vi "WPI_GyroClose.vi"(8 "error in (no error)":errorcluster, 11 "GyroDevRef":T1={"DevStatus"={"status"=FALSE, "code"=0, "source"=""}, "Analog Channel"=enum."AI 1", "Gain (VoltsPerDegree/Second)"=0.0, "Gyro Type"=enum."Analog", "Handle"=0, "SPI Bus"=enum."Invalid", "Device Found"=FALSE, "Sample Rate"=1.0, "Calibrate On Open"=FALSE, "Offset"=0.0} {"Sample Rate" min=0.25 max=100.0 step=0.25}) -> (0 "error out":errorcluster)   [LabVIEW 2017]
doc: "Closes the reference to the gyroscope you specify. Use this VI to close each gyroscope reference that you open with the Open VI.\n\nThis software is licensed. Open the labview\\readme\\WPI Robotics Library Open Source License.txt file for more information."
uses:
  <vilib>/Rock Robotics/WPI/Gyro/WPI_GyroDevRef.ctl
  <vilib>/Rock Robotics/SystemInterfaces/AI/FPGA_AIChannel.ctl
  <vilib>/Rock Robotics/SystemInterfaces/spilib/spi_bus.ctl
  <vilib>/Rock Robotics/SystemInterfaces/AI/FPGA_AIGyroChannel.ctl
  <instrlib>/Sparkfun Atomic IMU/HAIOL/Sparkfun Atomic IMU.lvclass
  <instrlib>/Honeywell Compass HMC6343/HAIOL/Honeywell Compass HMC6343.lvclass
panel:
  # "Analog"
  # "XRS"
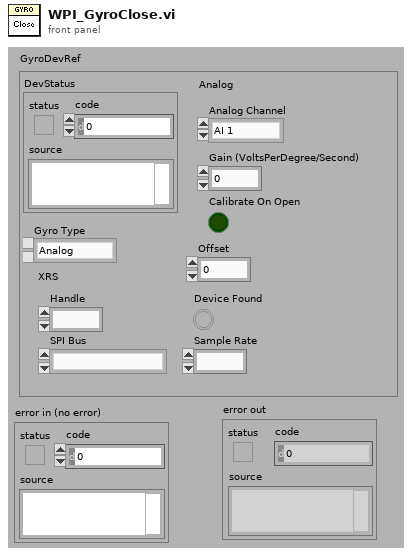
[diagram p1: front panel]
types:
  T1 = typedef "WPI_GyroDevRef.ctl" = cluster{"DevStatus":errorcluster, "Analog Channel":T2, "Gain (VoltsPerDegree/Second)":dbl, "Gyro Type":enum16{"Analog", "XRS450"}, "Handle":i32, "SPI Bus":T3, "Device Found":bool, "Sample Rate":dbl, "Calibrate On Open":bool, "Offset":dbl}
  T2 = typedef "FPGA_AIChannel.ctl" = enum8{"AI 0", "AI 1", "AI 2", "AI 3", "AI MXP 0", "AI MXP 1", "AI MXP 2", "AI MXP 3", "Invalid"}
  T3 = typedef "spi_bus.ctl" = enum16{"SPI On-Board, CS0", "SPI On-Board, CS1", "SPI On-Board, CS2", "SPI On-Board, CS3", "SPI MXP", "Invalid"}
  T4 = typedef "WPI_AnalogChannelDevRef.ctl" = cluster{"DevStatus":errorcluster, "Analog Channel":T2}
  T5 = typedef "FPGA_AIGyroChannel.ctl" = enum8{"AI 0", "AI 1", "Invalid"}
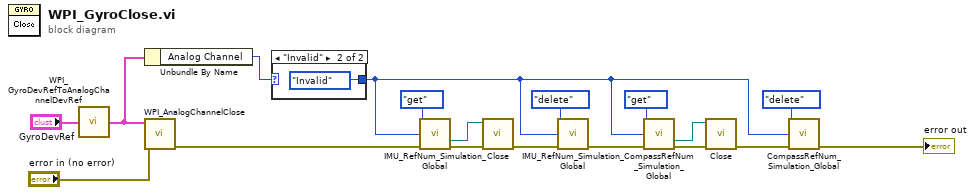
[diagram p0: block diagram]
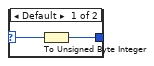
[diagram p2: hidden frame]
diagram:
  n1 = call <vilib>:"WPI_GyroDevRefToAnalogChannelDevRef.vi"("GyroDeviceRef"="GyroDevRef") -> ("AIDeviceRef"=w14:T4)  [unwired: 4 out]
  n2 = Unbundle By Name(w14) -> ("Analog Channel"=w13:T2)
  n3 = call <vilib>:"WPI_AnalogChannelClose.vi"("error in (no error)"="error in (no error)", "AIDeviceRef"=w14) -> ("error out"=w12:errorcluster)  [unwired: 9 out]
  n4 = case shown="\"Invalid\"" w13 {
    selector: w13 -> [w20 _]
    tunnel: [w19 FPGA_AIGyroChannel."Invalid" ("Analog Channel")] -> w3
    frame Default {
      n5 = To Unsigned Byte Integer(number=w20) -> (unsigned 8bit integer=w19:u8)
    }
    frame "Invalid" {
    }
  }
  n6 = call <vilib>:"IMU_RefNum_Simulation_Global.vi"("menu"=enum16{"set", "get", "delete"}."get", "Analog Channel"=w3, "error in (no error)"=w12) -> ("Sparkfun Atomic IMU Get"=w10:refnum<class "Sparkfun Atomic IMU.lvclass">, "error out"=w11:errorcluster)  [unwired: 11 in]
  n7 = call-dynamic "Close.vi"("error in (no error)"=w11, "Sparkfun Atomic IMU in"=w10) -> ("error out"=w8:errorcluster)  [unwired: 9 in]
  n8 = call <vilib>:"IMU_RefNum_Simulation_Global.vi"("menu"=enum16{"set", "get", "delete"}."delete", "Analog Channel"=w3, "error in (no error)"=w8) -> ("error out"=w7:errorcluster)  [unwired: 11 in, 1 out]
  n9 = call <vilib>:"CompassRefNum_Simulation_Global.vi"("menu"=enum16{"set", "get", "delete"}."get", "Analog Channel"=w3, "error in (no error)"=w7) -> ("Honeywell Compass HMC6343 Get"=w5:refnum<class "Honeywell Compass HMC6343.lvclass">, "error out"=w6:errorcluster)  [unwired: 11 in]
  n10 = call-dynamic "Close.vi"("error in (no error)"=w6, "Honeywell Compass HMC6343"=w5) -> ("error out"=w2:errorcluster)  [unwired: 9 in]
  n11 = call <vilib>:"CompassRefNum_Simulation_Global.vi"("menu"=enum16{"set", "get", "delete"}."delete", "Analog Channel"=w3, "error in (no error)"=w2) -> ("error out"=→"error out":errorcluster)  [unwired: 11 in, 1 out]
